vi "C4Hdl_getInterfaceName.vi"(0 "c4hdl in":refnum<k24>, 5 "ifNo in":i64, 11 "error in (no error)":errorcluster) -> (4 "c4hdl out":refnum<k24>, 6 "interface name out":string, 15 "error out":errorcluster)   [LabVIEW 2015, in "libC4HdlLV.lvlib"]
uses:
  libC4HdlLV.lvlib
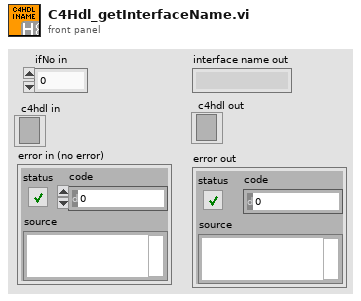
[diagram p1: front panel]
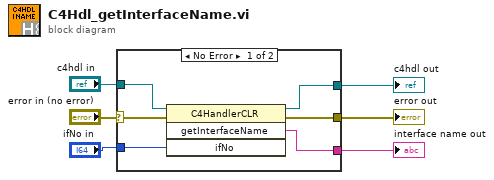
[diagram p0: block diagram]
diagram:
  n1 = case shown="No Error" "error in (no error)" {
    selector: "error in (no error)" -> [w10 w14]
    tunnel: [w12 w14] -> w6
    tunnel: [w11 w13] -> w5
    tunnel: "c4hdl in" -> [w9 w13]
    tunnel: [w8 _] -> w2
    tunnel: "ifNo in" -> [w7 _]
    frame No Error {
      n2 = invoke class="C4HandlerCLR" method="getInterfaceName"(reference=w9, error in=w10, "ifNo"=w7) -> (reference out=w11:refnum<k24>, error out=w12:errorcluster, "getInterfaceName"=w8:string)  [unwired: 1 in, 1 out]
    }
    frame Error {
    }
  }
  "error out" <- w6
  "c4hdl out" <- w5
  "interface name out" <- w2
